vi "Resize Unbundler.vi"(6 "Names":string[](array[string]), 8 "error in (no error)":errorcluster, 11 "VI in":refnum<vi>) -> (0 "error out":errorcluster, 2 "Unbundler Terminals":refnum<vi>[](array[refnum]), 3 "VI":refnum<vi>)   [LabVIEW 2020, in "Conditum-Tools.lvlib" / "Entity Editor.lvclass"]
uses:
  Entity Editor.lvclass
  <vilib>/Utility/traverseref.llb/TRef TravTarget.ctl
  <vilib>/Utility/traverseref.llb/VI Scripting - Traverse.lvlib
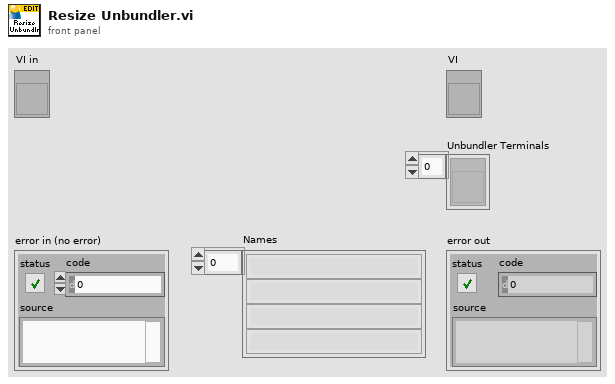
[diagram p1: front panel]
types:
  T1 = typedef "TRef TravTarget.ctl" = enum16{"FP", "BD", "Other"}
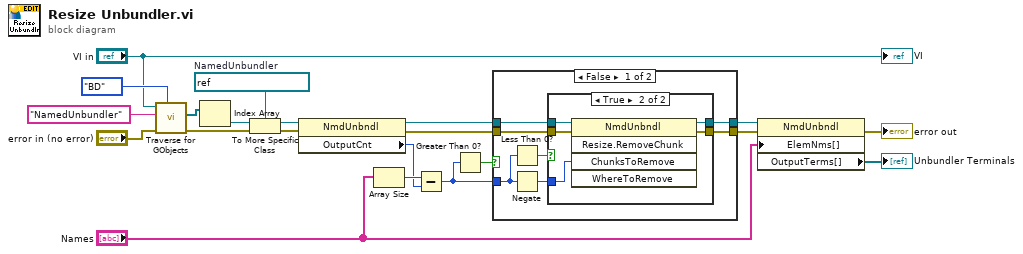
[diagram p0: block diagram]
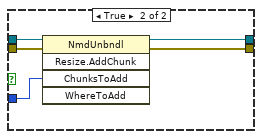
[diagram p3: hidden frame]
diagram:
  w18 = refnum<vi> refnum  # NamedUnbundler
  n1 = call <vilib>:"Traverse for GObjects.vi"("Traverse Target"=TRef_TravTarget."BD", "error in (no error)"="error in (no error)", "Class Name"="NamedUnbundler", "VI Refnum"="VI in") -> ("error out"=w17:errorcluster, "References"=w20:refnum<vi>[])  [unwired: 4 in, 2 out]
  n2 = Index Array(array=w20) -> (element=w19:refnum<vi>)  [unwired: 1 in]
  n3 = To More Specific Class(target class=w18, reference=w19, error in=w17) -> (specific class reference=w15:refnum<vi>, error out=w16:errorcluster)
  n4 = property class="NmdUnbndl"(reference=w15, error in=w16) -> (reference out=w14:refnum<vi>, error out=w13:errorcluster, "OutputCnt"=w1:i32)
  n5 = Array Size(array="Names") -> (size(s)=w12:i32)
  n6 = Subtract(x=w12, y=w1) -> (x-y=w11:i32)
  n7 = Greater Than 0?(x=w11) -> (x > 0?=w10:bool)
  n8 = case shown="False" w10 {
    tunnel: w14 -> [w26 w40]
    tunnel: w13 -> [w25 w39]
    tunnel: w11 -> [w27 w38]
    tunnel: [w24 w37] -> w9
    tunnel: [w23 w36] -> w8
    frame False {
      n9 = Less Than 0?(x=w27) -> (x < 0?=w28:bool)
      n10 = Negate(x=w27) -> (-x=w22:i32)
      n11 = case shown="True" w28 {
        tunnel: w22 -> [_ w33]
        tunnel: w26 -> [w30 w35]
        tunnel: w25 -> [w29 w34]
        tunnel: [w30 w32] -> w24
        tunnel: [w29 w31] -> w23
        frame False {
        }
        frame True {
          n12 = invoke class="NmdUnbndl" method="Resize.RemoveChunk"(reference=w35, error in=w34, "ChunksToRemove"=w33) -> (reference out=w32:refnum<vi>, error out=w31:errorcluster)  [unwired: 2 in, 3 out]
        }
      }
    }
    frame True {
      n13 = invoke class="NmdUnbndl" method="Resize.AddChunk"(reference=w40, error in=w39, "ChunksToAdd"=w38) -> (reference out=w37:refnum<vi>, error out=w36:errorcluster)  [unwired: 2 in, 3 out]
    }
  }
  n14 = property class="NmdUnbndl"(reference=w9, error in=w8, "ElemNms[]"="Names") -> (error out=→"error out":errorcluster, "OutputTerms[]"=→"Unbundler Terminals":refnum<vi>[])  [unwired: 1 out]
  "VI" <- "VI in"
